vi "LAbo2.2.vi"() -> ()   [LabVIEW 2020]
panel:
  out "Wartosc logiczna na koncu 2":bool
  out "Wartosc logiczna na koncu":bool
  in  "stop":bool
  out "String 2":string
  in  "wrtoœæ logiczna q: 2":bool
  in  "wrtoœæ logiczna p: 2":bool
  out "String":string
  in  "wrtoœæ logiczna q:":bool
  in  "wrtoœæ logiczna p:":bool
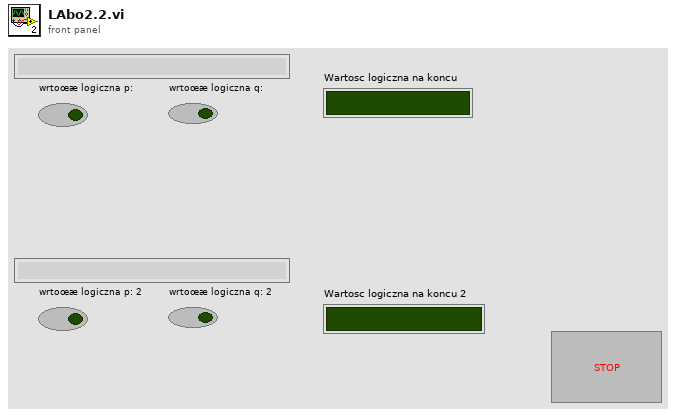
[diagram p1: front panel]
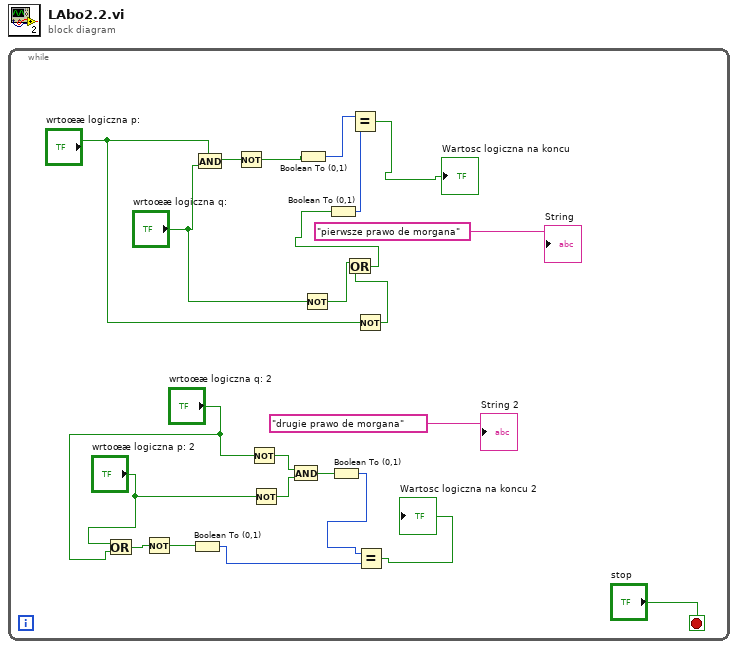
[diagram p0: block diagram]
diagram:
  n1 = while {
    stop <- "stop" stop-if-true
    n2 = Or(x="wrtoœæ logiczna p: 2", y="wrtoœæ logiczna q: 2") -> (x .or. y?=w8:bool)
    n3 = Not(x=w8) -> (.not. x?=w7:bool)
    n4 = Boolean To (0,1)(Boolean=w7) -> (0, 1=w6:i16)
    n5 = And(x="wrtoœæ logiczna p:", y="wrtoœæ logiczna q:") -> (x .and. y?=w21:bool)
    n6 = Not(x=w21) -> (.not. x?=w20:bool)
    n7 = Not(x="wrtoœæ logiczna q: 2") -> (.not. x?=w13:bool)
    n8 = Not(x="wrtoœæ logiczna p: 2") -> (.not. x?=w12:bool)
    n9 = And(x=w13, y=w12) -> (x .and. y?=w11:bool)
    n10 = Boolean To (0,1)(Boolean=w20) -> (0, 1=w23:i16)
    n11 = Not(x="wrtoœæ logiczna q:") -> (.not. x?=w17:bool)
    n12 = Boolean To (0,1)(Boolean=w11) -> (0, 1=w10:i16)
    n13 = Not(x="wrtoœæ logiczna p:") -> (.not. x?=w1:bool)
    n14 = Or(x=w17, y=w1) -> (x .or. y?=w16:bool)
    n15 = Boolean To (0,1)(Boolean=w16) -> (0, 1=w22:i16)
    n16 = Equal?(x=w23, y=w22) -> (x = y?=→"Wartosc logiczna na koncu":bool)
    n17 = Equal?(x=w10, y=w6) -> (x = y?=→"Wartosc logiczna na koncu 2":bool)
    "String" <- "pierwsze prawo de morgana"
    "String 2" <- "drugie prawo de morgana"
  }
